vi "remaining_string.vi"() -> ()   [LabVIEW 2011]
panel:
  in  "remaining string":string
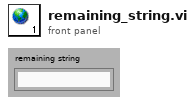
[diagram p1: front panel]
diagram:
